vi "DoDone Sandbox.vi"() -> ()   [LabVIEW 2019]
panel:
  out "Done":bool
  in  "Do":bool
  in  "Init":bool
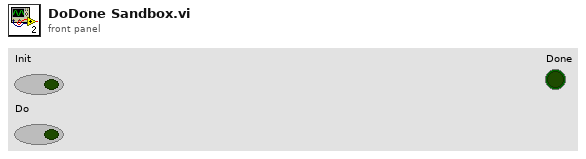
[diagram p1: front panel]
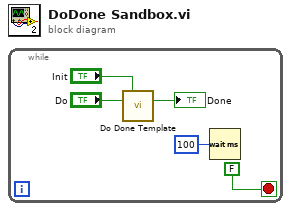
[diagram p0: block diagram]
diagram:
  n1 = while {
    stop <- FALSE stop-if-true
    n2 = call "Do Done Template.vi"("Init"="Init", "Do"="Do") -> ("Done"=→"Done":bool)  [unwired: 13 in]
    n3 = Wait (ms)(milliseconds to wait=u32 100) -> ()  [unwired: 1 out]
  }
